vi "SIM Eval Error.vi"(0 "Solution":dbl[](array[numeric]), 1 "relative tolerance":dbl, 2 "absolute tolerance":dbl, 3 "min float":dbl, 5 "estimated error":dbl[](array[numeric]), 7 "max step size":dbl, 9 "max step ratio":dbl, 11 "proposed step size":dbl, 12 "step size":dbl, 13 "min step size":dbl, 14 "error order":i32) -> (4 "Solution Out":dbl[](array[numeric]), 6 "proposed step size out":dbl, 8 "new step size ratio":dbl, 10 "step accepted?":bool)   [LabVIEW 2020]
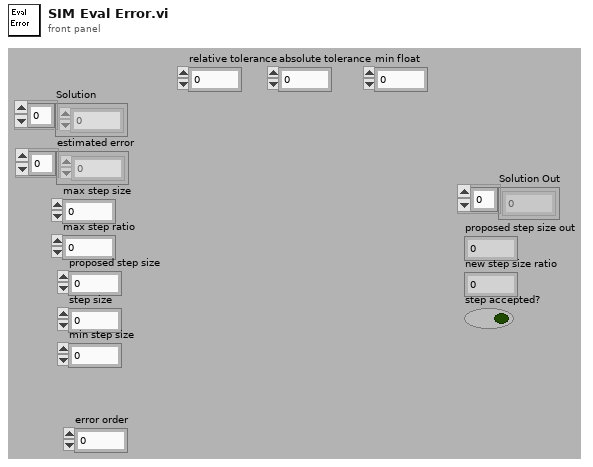
[diagram p1: front panel]
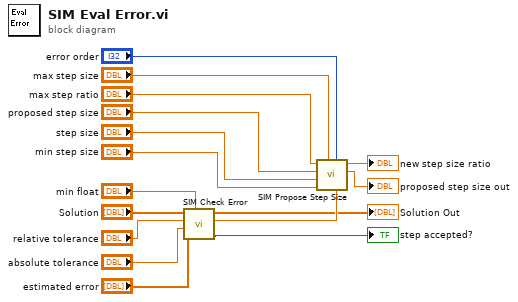
[diagram p0: block diagram]
diagram:
  n1 = call "SIM Check Error.vi"("min float"="min float", "estimated error"="estimated error", "absolute tolerance"="absolute tolerance", "relative tolerance"="relative tolerance", "Solution"="Solution") -> ("within acceptable err?"=→"step accepted?":bool, "acceptable err/estimated err"=w2:dbl, "Solution Out"=→"Solution Out":dbl[])  [unwired: 1 in, 3 out]
  n2 = call "SIM Propose Step Size.vi"("acceptable err/estimated err"=w2, "error order"="error order", "max step size"="max step size", "min step size"="min step size", "step size"="step size", "proposed step size"="proposed step size", "max step ratio"="max step ratio") -> ("proposed step size out"=→"proposed step size out":dbl, "proposed max step ratio"=→"new step size ratio":dbl)  [unwired: 3 out]
